vi "modbus.vi"(0 "VISA resource name for Modbus":refnum<visa-resource-name>="COM5", 1 "起始地址ADR低位":string="00") -> (2 "read buf":string, 3 "通信指示":bool, 4 "error out":errorcluster={"status"=FALSE, "code"=1073676294, "source"="modbus.vi中的VISA读取"})   [LabVIEW 2012]
uses:
  <vilib>/Instr/_visa.llb/VISA Configure Serial Port (Instr).vi
panel:
  out "element":u8=2
  out "unsigned byte array":u8[](array[numeric])=[1, 3, 2, 0, 2, 57, 133]
  out "结果":string
  in  "数据数目高位":string="00"
  in  "起始地址ADR高位":string="00"
  in  "数据数目低位":string="01"
  in  "命令码 CMD":string="03"
  in  "通讯地址ADR":string="01"
  # "01"
  # "01"
  # "00"
  # "00"
  # "00"
  # "08"
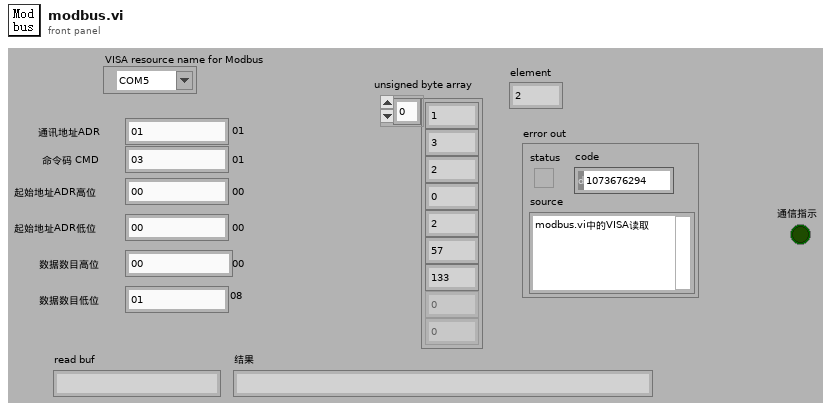
[diagram p1: front panel]
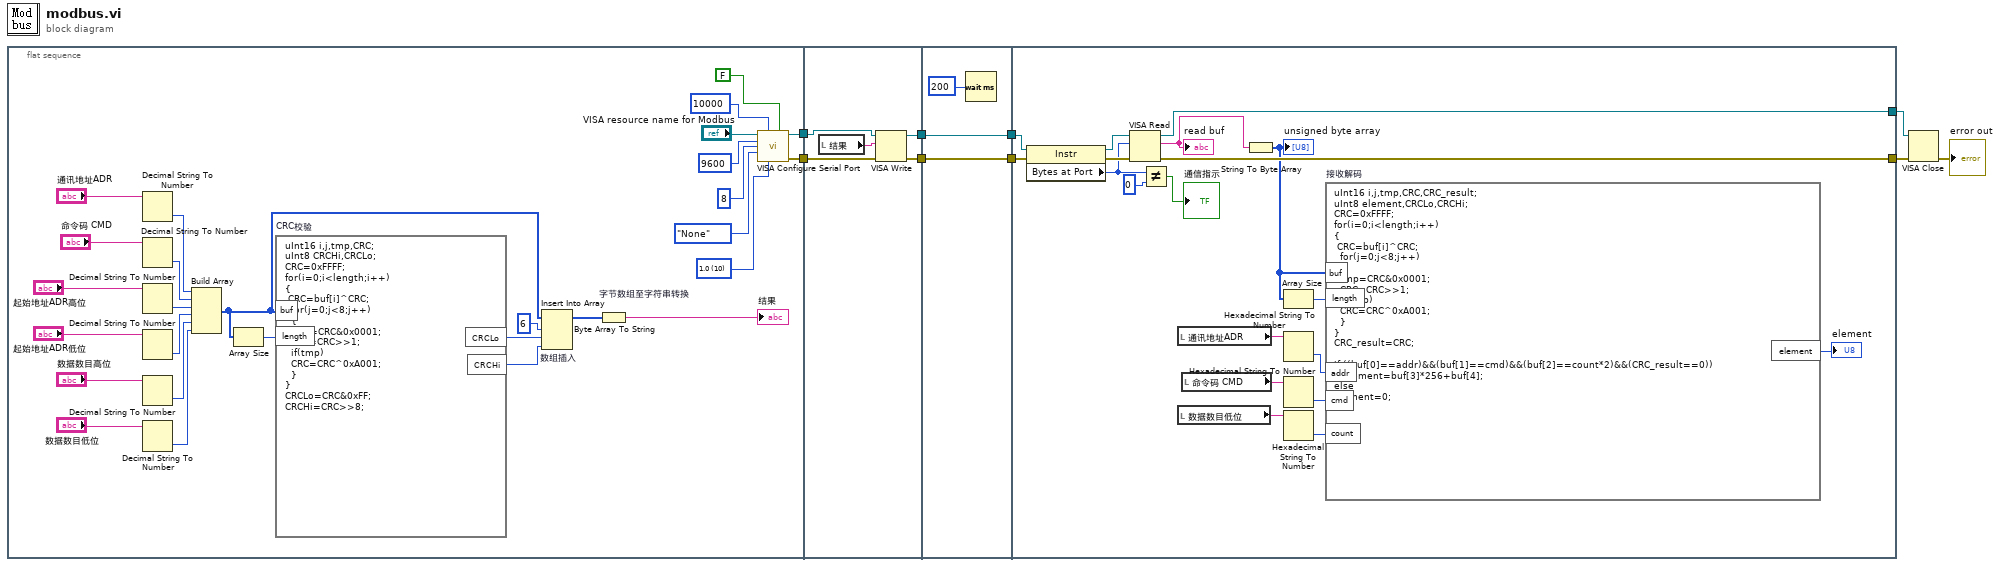
[diagram p0: block diagram]
diagram:
  n1 = flat-sequence {
    tunnel: [w31] -> w2
    tunnel: [w30] -> w1
    tunnel: [w42] -> w6
    tunnel: [w41] -> w5
    tunnel: w2 -> [w40]
    tunnel: w1 -> [w38]
    tunnel: w6 -> [w44]
    tunnel: [w44] -> w4
    tunnel: w5 -> [w43]
    tunnel: [w43] -> w3
    tunnel: w4 -> [w62]
    tunnel: w3 -> [w61]
    tunnel: [w60] -> w7
    tunnel: [w59] -> w8
    frame #0 {
      w36 = u16 10 items=["1.0"=10, "1.5"=15, "2.0"=20] ("stop bits (10: 1 bit)")
      n2 = Decimal String To Number(string="通讯地址ADR") -> (number=w12:i32)  [unwired: 2 in, 1 out]
      n3 = Decimal String To Number(string="命令码 CMD") -> (number=w11:i32)  [unwired: 2 in, 1 out]
      n4 = Decimal String To Number(string="起始地址ADR高位") -> (number=w25:i32)  [unwired: 2 in, 1 out]
      n5 = Decimal String To Number(string="起始地址ADR低位") -> (number=w26:i32)  [unwired: 2 in, 1 out]
      n6 = Decimal String To Number(string="数据数目高位") -> (number=w27:i32)  [unwired: 2 in, 1 out]
      n7 = Decimal String To Number(string="数据数目低位") -> (number=w28:i32)  [unwired: 2 in, 1 out]
      n8 = Build Array(w12, w11, w25, w26, w27, w28) -> (w20:i32[])
      n9 = Array Size(array=w20) -> (size(s)=w19:i32)
      n10 = formula code="uInt16 i,j,tmp,CRC;\nuInt8 CRCHi,CRCLo;\nCRC=0xFFFF;\nfor(i=0;i<length;i++)\n{\n CRC=buf[i]^CRC;\n  for(j=0;j<8;j++)\n  {\n  tmp=CRC&0x0001;\n  CRC=CRC>>1;\n  if(tmp)\n  CRC=CRC^0xA001;\n  }\n}\nCRCLo=CRC&0xFF;\nCRCHi=CRC>>8;" "CRC校验"("buf"=w20, "length"=w19) -> ("CRCLo"=w22:u8, "CRCHi"=w21:u8)
      n11 = Insert Into Array "数组插入"(array=w20, index=6, new element #1=w22, new element #2=w21) -> (w23:i32[])
      n12 = Byte Array To String "字节数组至字符串转换"(unsigned byte array=w23) -> (string=→"结果":string)
      n13 = call-poly "VISA Configure Serial Port"("VISA resource name"="VISA resource name for Modbus", "timeout (10sec)"=u32 10000, "Enable Termination\nChar (T)"=FALSE ("Enable Termination\nChar (T)"), "baud rate (9600)"=u32 9600, "data bits (8)"=u16 8, "parity (0:none)"=enum16{"None", "Odd", "Even", "Mark", "Space"}."None", "stop bits (10: 1 bit)"=w36) -> ("VISA resource name out"=w31:refnum<visa-resource-name>, "error out"=w30:errorcluster)  [unwired: 7 in]
    }
    frame #1 {
      n14 = local read "结果"() -> (w39:string)
      n15 = VISA Write(VISA resource name=w40, write buffer=w39, error in (no error)=w38) -> (VISA resource name out=w41:refnum<visa-resource-name>, error out=w42:errorcluster)  [unwired: 1 out]
    }
    frame #2 {
      n16 = Wait (ms)(milliseconds to wait=u32 200) -> ()  [unwired: 1 out]
    }
    frame #3 {
      n17 = property class="Instr"(reference=w61, error in=w62) -> (reference out=w64:refnum<visa-resource-name>, error out=w63:errorcluster, "Bytes at Port"=w47:u32)
      n18 = VISA Read(VISA resource name=w64, byte count=w47, error in (no error)=w63) -> (VISA resource name out=w59:refnum<visa-resource-name>, read buffer=w49:string, error out=w60:errorcluster)  [unwired: 1 out]
      "read buf" <- w49
      n19 = Not Equal?(x=w47, y=u32 0) -> (x != y?=→"通信指示":bool)
      n20 = local read "通讯地址ADR"() -> (w56:string)
      n21 = local read "数据数目低位"() -> (w51:string)
      n22 = local read "命令码 CMD"() -> (w52:string)
      n23 = String To Byte Array(string=w49) -> (unsigned byte array=w54:u8[])
      "unsigned byte array" <- w54
      n24 = Array Size(array=w54) -> (size(s)=w58:i32)
      n25 = Hexadecimal String To Number(string=w56) -> (number=w57:u32)  [unwired: 2 in, 1 out]
      n26 = Hexadecimal String To Number(string=w52) -> (number=w55:u32)  [unwired: 2 in, 1 out]
      n27 = Hexadecimal String To Number(string=w51) -> (number=w50:u32)  [unwired: 2 in, 1 out]
      n28 = formula code="uInt16 i,j,tmp,CRC,CRC_result;\nuInt8 element,CRCLo,CRCHi;\nCRC=0xFFFF;\nfor(i=0;i<length;i++)\n{\n CRC=buf[i]^CRC;\n  for(j=0;j<8;j++)\n  {\n  tmp=CRC&0x0001;\n  CRC=CRC>>1;\n  if(tmp)\n  CRC=CRC^0xA001;\n  }\n}\nCRC_result=CRC;\n\nif ((buf[0]==addr)&&(buf[1]==cmd)&&(buf[2]==count*2)&&(CRC_result==0))\n   element=buf[3]*256+buf[4];\nelse\nelement=0;" "接收解码"("buf"=w54, "length"=w58, "addr"=w57, "cmd"=w55, "count"=w50) -> ("element"=→"element":u8)
    }
  }
  n29 = VISA Close(VISA resource name=w8, error in (no error)=w7) -> (error out=→"error out":errorcluster)
